vi "Calculate_Velocity.vi"(2 "Times":T1 {"Accelation fractional distance" format="%.2f"; "Accelaration time" format="%.7f"; "Total travel time" format="%.7f"}, 5 "Revs to travel":dbl format="%.2f") -> (0 "Acceleration":dbl format="%.2f", 1 "Max Velocity":dbl format="%.2f")   [LabVIEW 2010]
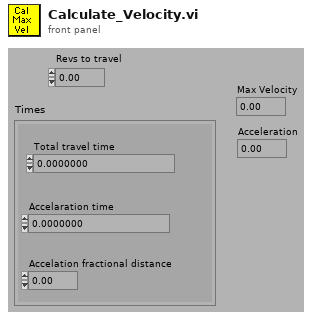
[diagram p1: front panel]
types:
  T1 = cluster{"Total travel time":dbl, "Accelaration time":dbl, "Accelation fractional distance":dbl}
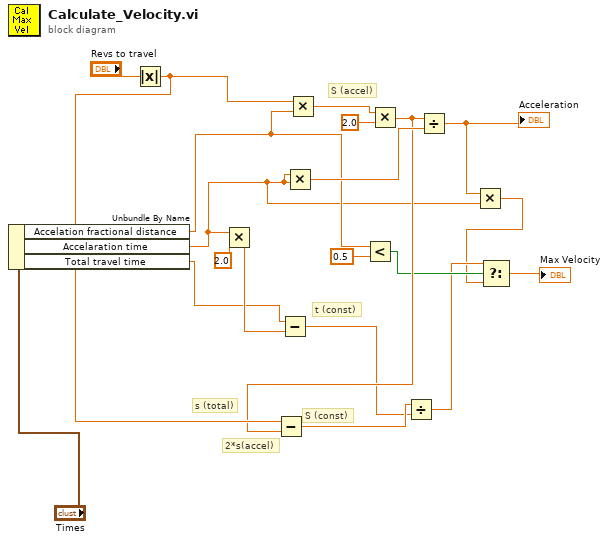
[diagram p0: block diagram]
diagram:
  # "t (const)"
  # "S (const)"
  # "s (total)"
  # "2*s(accel)"
  # "S (accel)"
  n1 = Unbundle By Name("Times") -> ("Accelation fractional distance"=w2:dbl, "Accelaration time"=w1:dbl, "Total travel time"=w3:dbl)
  n2 = Absolute Value(x="Revs to travel") -> (abs(x)=w14:dbl)
  n3 = Multiply(x=w1, y=2.0) -> (x*y=w15:dbl)
  n4 = Subtract(x=w3, y=w15) -> (x-y=w11:dbl)
  n5 = Multiply(x=w1, y=w1) -> (x*y=w17:dbl)
  n6 = Multiply(x=w14, y=w2) -> (x*y=w19:dbl)
  n7 = Less?(x=w2, y=0.5) -> (x < y?=w9:bool)
  n8 = Multiply(x=w19, y=2.0) -> (x*y=w13:dbl)
  n9 = Subtract(x=w14, y=w13) -> (x-y=w12:dbl)
  n10 = Divide(x=w12, y=w11) -> (x/y=w8:dbl)
  n11 = Divide(x=w13, y=w17) -> (x/y=w6:dbl)
  "Acceleration" <- w6
  n12 = Multiply(x=w6, y=w1) -> (x*y=w5:dbl)
  n13 = Select(t=w8, s=w9, f=w5) -> (s? t:f=→"Max Velocity":dbl)
